vi "Get_Weld_History_Repeated_webserver.vi"() -> ()   [LabVIEW 2017]
uses:
  Generic_Common/Webserver/html_report_cluster.ctl
  <vilib>/httpClient/LabVIEWHTTPClient.lvlib
panel:
  out "vi path":path
  out "Fail":picture
  out "Pass":picture
  out "Iteration Status":bool[](array[boolean])
  out "Grobal Status":bool
  out "Global path":path
  out "Local ini path":path
  out "filename":string
  out "Results Path":path
  in  "Iterations":i32 caption="Iterations (0 to finish:)" min=0
  in  "Resume":bool
  out "error out":errorcluster
  out "key":string
  out "password":string
  out "userid":string
  out "login_url":string
  in  "Delay (ms):":i32
  out "StatusCodeName":string
  out "Session id name":string
  out "logout_url":string
  out "ErrorCode_expected":string
  out "Logout : Header  debug purpose":string
  out "Logout : Body debug purpose":string
  out "Status_message":string
  out "Logo":u16(ring)
  out "Iteration_Indicator":i32
  out "Error code recieved":i32
  out "POST_command":string
  out "Command_url":string
  out "Test case":string
  out "Global ini path":path
  out "Test status":picture
  out "Time elapsed for each iteration":string
  out "DelayBetweenIterations":string
  out "Global_Webserver_Report":string
  out "TestSuite":string
  out "Error Out":errorcluster
  out "Response time":u32[](graph)
  out "Header of reponse for debug pupose":string
  out "Response":string caption="Response from the web server"
  # "AUTOMATION TESTING WEB SERVICES"
  # "TESTING DETAILS FROM INI"
  # "RESPONSE FROM WEBSERVER"
  # "ms"
  # "Webserver \n1. Webserver is being tested in this test case where SC board of ultrasonic welding machine is connected to test PC \t\t  \nSC IP address: 192.168.2.101, url=https://192.168.2.101\t\t\t\t\t\t\t\t\t\t \t\t\t  \n2. Ports used on SC board are as below:\t\t\t\t\t\t\t\t\t\t\t\t\t\t\t\t\t\t\t\t\t  \n   - J103: (Ethernet0) This port connected to UI controller large screen HMI display\trestricted webservices in this port\t\t\t\t\t\t\t\t\t  \n  - J104: (Ethernet1) This port is connected to local area network for accessing the webpage and testing  webserver                                \n  - J112: SC Logs are taken from this port. TeraTerm is configured  to this port so that SC logs are displayed on the screen."
  # "TESTING STATUS"
  # "RESPONSE TIME GRAPH"
  # "GLOBAL TESTING STATUS"
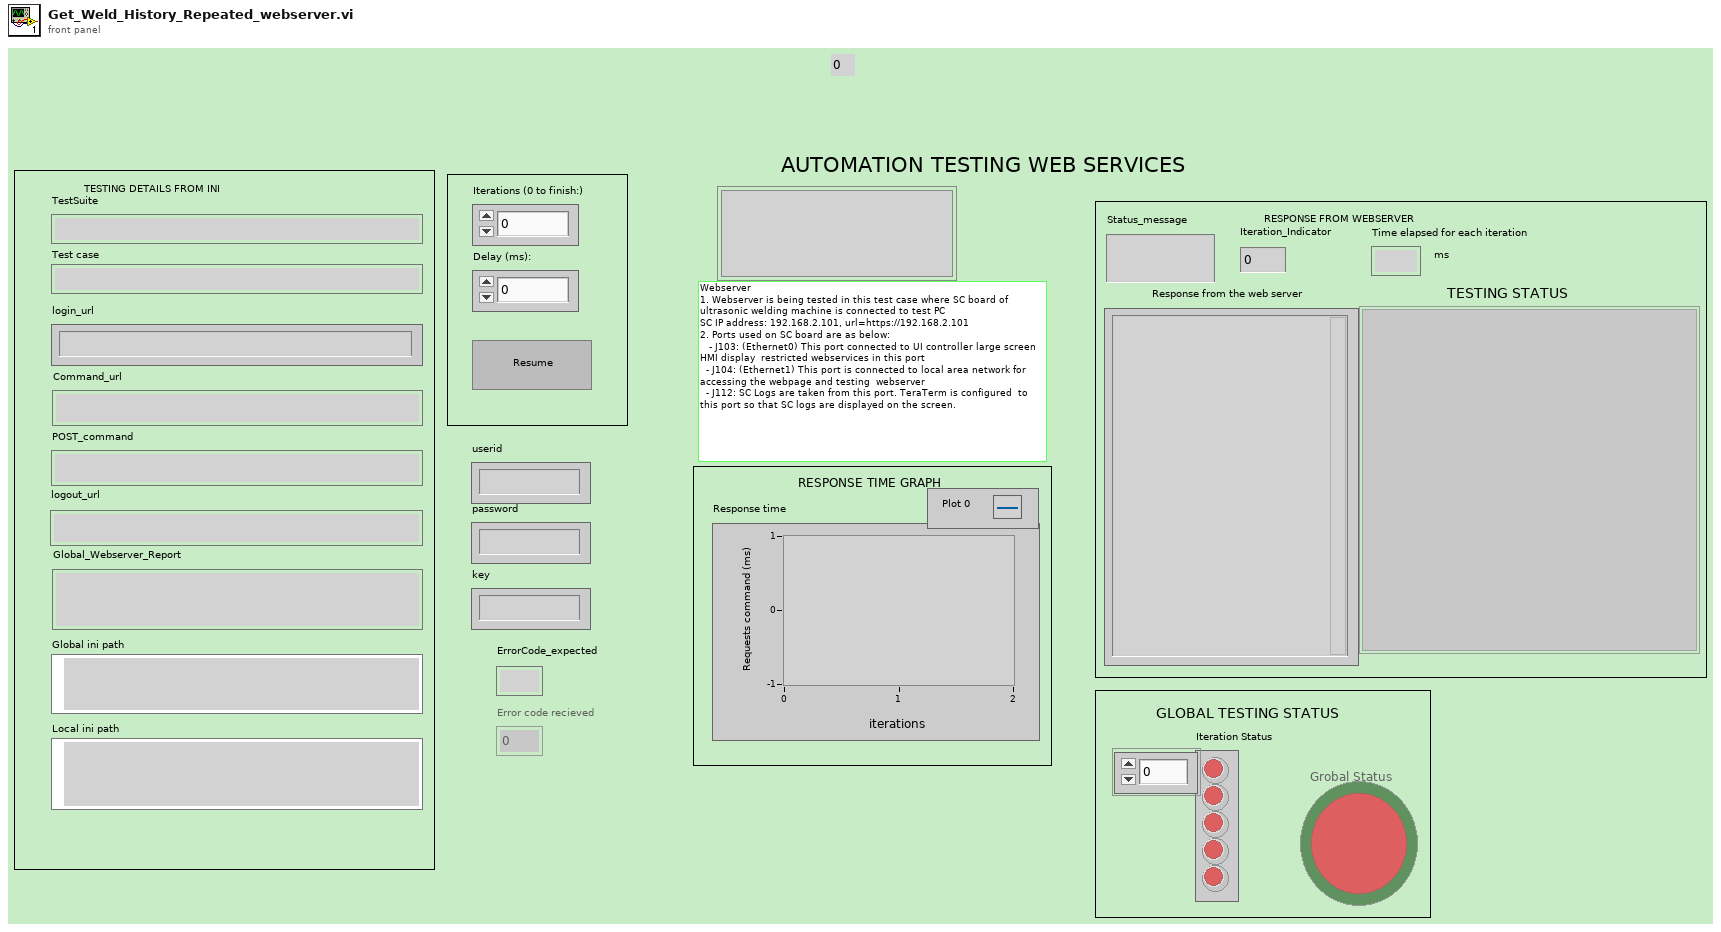
[diagram p1: front panel]
types:
  T1 = enum16{"open", "replace", "create", "open or create", "replace or create", "replace or create with confirmation"}
  T2 = enum8{"Enabled", "Disabled", "Disabled and Grayed Out"}
  T3 = typedef "imagedata.ctl" = cluster{"image type":i32, "image depth":i32, "image":u8[], "mask":u8[], "colors":u32[], "Rectangle":cluster{"left":i16, "top":i16, "right":i16, "bottom":i16}}
  T4 = cluster{"[0]":string, "[1]":string, "[2]":string, "[3]":string, "[4]":string, "[5]":string, "[6]":string, "[7]":string, "[8]":string}
  T5 = cluster{"Server_IP_Address":string, "Server_Port_Number":string, "Sid":string, "StatusCodeName":string, "Global_Webserver_Report":string}
  T6 = cluster{"login_url":string, "userid":string, "password":string, "key":string, "command_url":string, "POST_command":string, "StatusCode_expected":string, "Iterations":string, "DelayBetweenIterations":string, "Timeout":string, "logout_url":string}
  T7 = typedef "html_report_cluster.ctl" = cluster{"Remarks":string, "Verdict":string, "Status Code":i32, "Status Description":string, "JazzDashboardLink":string, "ReprtPath":string, "Timestamp":string, "TestSuite":string, "TestCase":string, "Iterations":i64, "Time taken to execute  test in msec":string, "Delay Between Iterations":i64}
  T8 = typedef "LabVIEWHTTPClient.lvlib/ClientHandle.ctl" = refnum<k1>
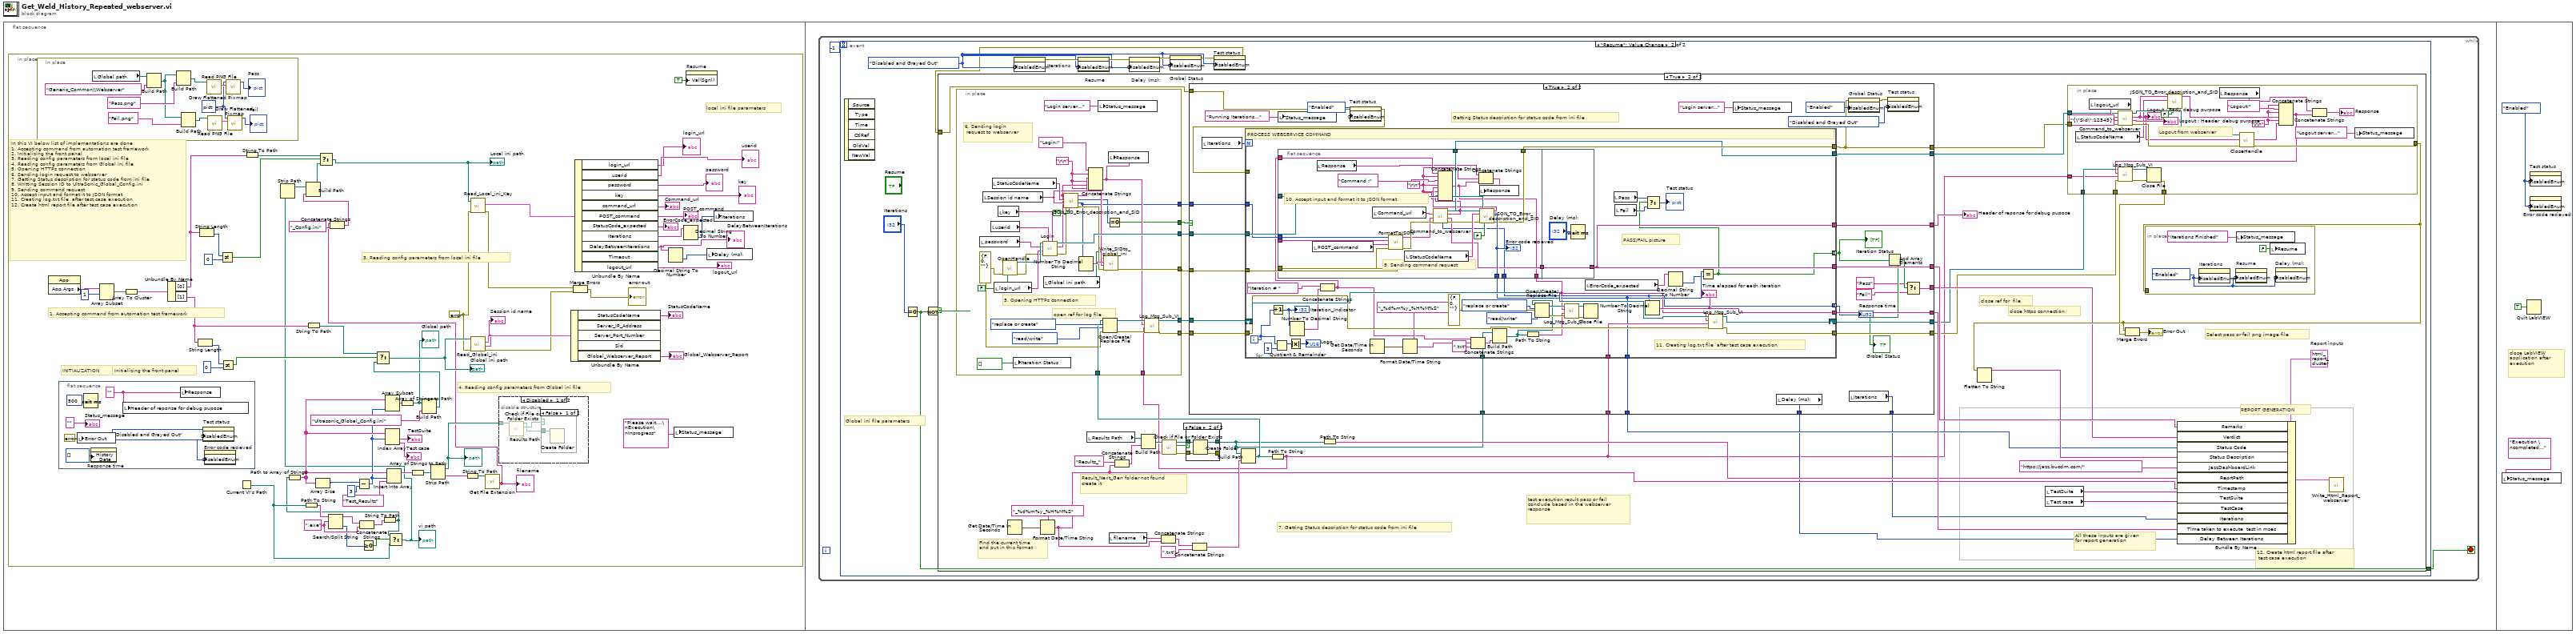
[diagram p0: block diagram]
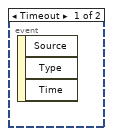
[diagram p4: hidden frame]
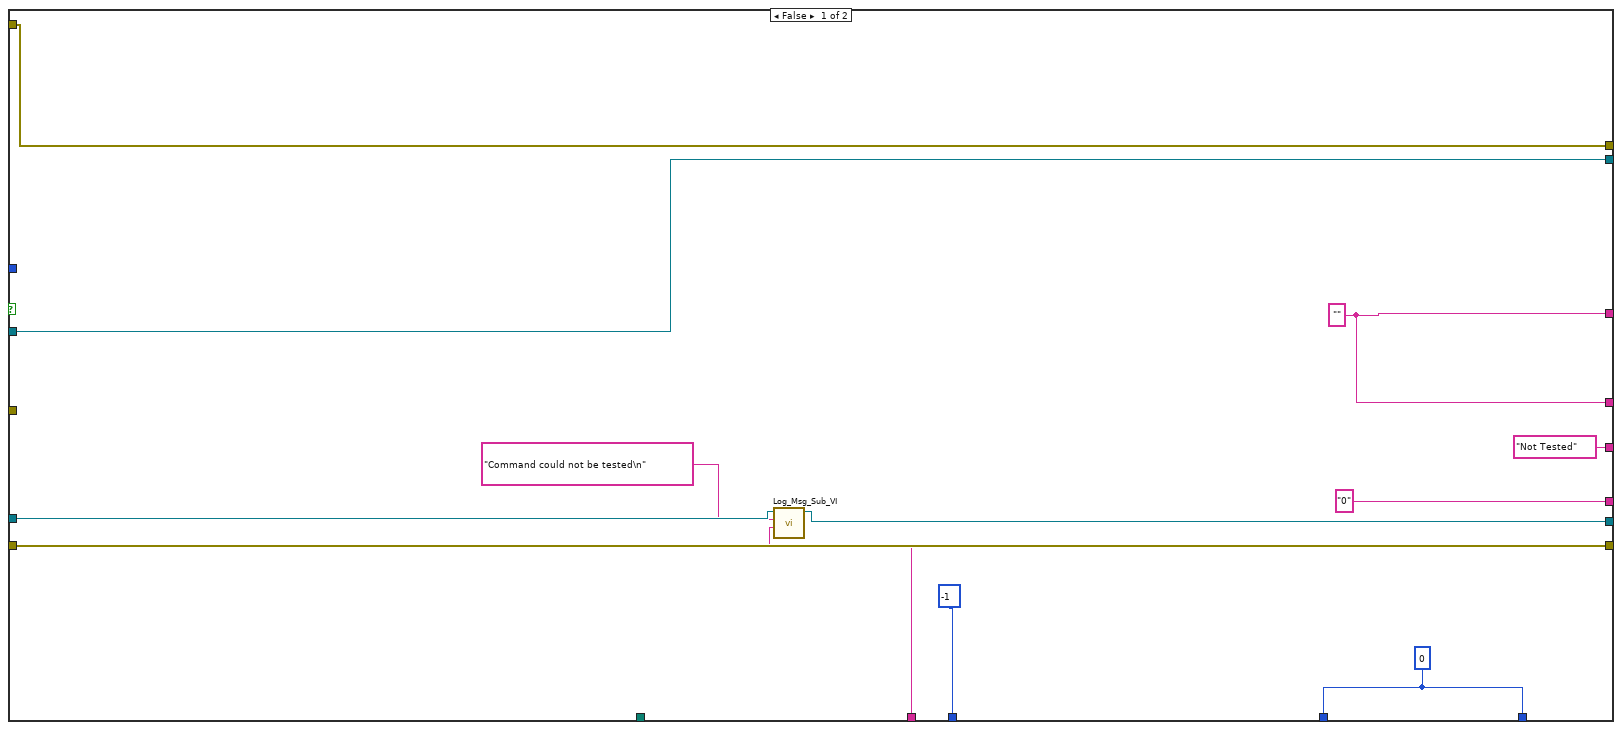
[diagram p6: hidden frame]
diagram:
  n1 = flat-sequence {
    frame #0 {
      n2 = in-place {
        w7 = ".exe" ("search string/char (-)")
        w21 = errorcluster {"status"=FALSE, "code"=0, "source"=""} ("error out")
        # "local ini file parameters"
        # "INITIALIZATION"
        # "4. Reading config parameters from Global ini file"
        # "3. Reading config parameters from local ini file"
        # "2. Initializing the front panel"
        # "1. Accepting command from automation test framework"
        # "In this VI below list of implementations are done\n1. Accepting command from automation test framework\n2. Initializing the front panel\n3. Reading config parameters from local ini file\n4. Reading config parameters from Global ini file\n5. Opening HTTPs connection\n6. Sending login request to webserver\n7. Getting Status description for status code from ini file\n8. Writting Session ID to UltraSonic_Global_Config.ini\n9. Sending command request\n10. Accept input and format it to JSON format\n11. Creating log.txt file  after test case execution\n12. Create html report file after test case execution"
        n3 = in-place {
          w70 = picture data[5B] ("picture")
          n4 = local read "Global path"() -> (w78:path)
          n5 = Build Path(base path=w78, name or relative path="Generic_Common\\Webserver") -> (appended path=w72:path)
          n6 = Build Path(base path=w72, name or relative path="Pass.png") -> (appended path=w76:path)
          n7 = Build Path(base path=w72, name or relative path="Fail.png") -> (appended path=w73:path)
          n8 = call <vilib>:"Read PNG File.vi"("path to PNG file"=w76) -> ("image data"=w80:T3)  [unwired: 8 in, 2 out]
          n9 = call <vilib>:"Read PNG File.vi"("path to PNG file"=w73) -> ("image data"=w75:T3)  [unwired: 8 in, 2 out]
          n10 = call <vilib>:"Draw Flattened Pixmap.vi"("image data"=w80, "picture"=w70) -> ("new picture"=→"Pass":picture)  [unwired: 7 in]
          n11 = call <vilib>:"Draw Flattened Pixmap.vi"("image data"=w75, "picture"=w70) -> ("new picture"=→"Fail":picture)  [unwired: 7 in]
        }
        n12 = property class="App"() -> ("App.Args"=w63:string[])  [unwired: 2 in, 2 out]
        n13 = flat-sequence {
          frame #0 {
            w86 = T2."Disabled and Grayed Out" ("Disabled")
            w91 = ""
            n14 = local write "Error Out"(errorcluster {"status"=FALSE, "code"=0, "source"=""} ("error constant")) -> ()
            n15 = Wait (ms)(milliseconds to wait=u32 500) -> ()  [unwired: 1 out]
            n16 = property on="Response time" class="WFChart (strict)"("History Data"=u32[] []) -> ()  [unwired: 2 in, 2 out]
            n17 = local write "Header of reponse for debug pupose"(w91) -> ()
            n18 = local write "Response"(w91) -> ()
            n19 = property on="Test status" class="Pict"("DisabledEnum"=w86) -> ()  [unwired: 2 in, 2 out]
            n20 = property on="Error code recieved" class="DigNum (strict)"("DisabledEnum"=w86) -> ()  [unwired: 2 in, 2 out]
            "Status_message" <- ""
          }
        }
        n21 = Array Subset "Array Subset"(array=w63, index=1) -> (w64:string[])  [unwired: 1 in]
        n22 = Array To Cluster(array=w64) -> (cluster=w65:T4)
        n23 = Unbundle By Name "Unbundle By Name"(w65) -> ("[0]"=w14:string, "[1]"=w15:string)
        n24 = String Length(string=w15) -> (length=w69:i32)
        n25 = String Length(string=w14) -> (length=w66:i32)
        n26 = Not Equal?(x=w66, y=0) -> (x != y?=w10:bool)
        n27 = Not Equal?(x=w69, y=0) -> (x != y?=w30:bool)
        n28 = Current VI's Path() -> (path=w3:path)
        n29 = String To Path(string=w14) -> (path=w17:path)
        n30 = Path To String(path=w3) -> (string=w9:string)
        n31 = String To Path(string=w15) -> (path=w29:path)
        n32 = Search/Split String(string=w9, search string/char (-)=w7) -> (substring before match=w8:string, offset of match=w4:i32)  [unwired: 1 in, 1 out]
        n33 = Concatenate Strings(w8, w7) -> (w6:string)
        n34 = Greater Or Equal To 0?(x=w4) -> (x >= 0?=w5:bool)
        n35 = String To Path(string=w6) -> (path=w2:path)
        n36 = Path to Array of Strings(0:w2) -> (2:w33:string[])  [unwired: 1 out]
        n37 = Array Size(array=w33) -> (size(s)=w41:i32)
        n38 = Subtract(x=w41, y=3) -> (x-y=w32:i32)
        n39 = Index Array(array=w33, index #1=w32) -> (element #1=→"TestSuite":string, element #2=→"Test case":string)  [unwired: 1 in]
        n40 = Array Subset(array=w33, length=w32) -> (w31:string[])  [unwired: 1 in]
        n41 = Insert Into Array(array=w33, index=w32, new element="Test_Results" ("new element/subarray")) -> (w39:string[])
        n42 = Select(t=w2, s=w5, f=w3) -> (s? t:f=w1:path)
        "vi path" <- w1
        n43 = Strip Path(path=w1) -> (stripped path=w18:path)  [unwired: 1 out]
        n44 = Array of Strings to Path(0:w31) -> (2:w12:path)  [unwired: 1 in]
        "Global path" <- w12
        n45 = Array of Strings to Path(0:w39) -> (2:w40:path)  [unwired: 1 in]
        n46 = Build Path(base path=w12, name or relative path="Ultrasonic_Global_Config.ini") -> (appended path=w23:path)
        n47 = Select(t=w29, s=w30, f=w23) -> (s? t:f=w28:path)
        "Global ini path" <- w28
        n48 = Strip Path(path=w40) -> (stripped path=w36:path, name=w37:string)
        "Results Path" <- w36
        n49 = String To Path(string=w37) -> (path=w38:path)
        n50 = call "Read_Global_ini.vi"("Error In"=w21, "Global ini path"=w28) -> ("Error Out"=w60:errorcluster, "Session id name"=→"Session id name":string, "Global Cluster"=w61:T5)  [unwired: 7 in]
        n51 = call <vilib>:"Get File Extension.vi"("file"=w38) -> ("filename without extension"=w11:string)  [unwired: 6 in, 4 out]
        "filename" <- w11
        n52 = Concatenate Strings(w11, "_Config.ini" ("element")) -> (w20:string)
        n53 = Build Path(base path=w18, name or relative path=w20) -> (appended path=w19:path)
        n54 = Select(t=w17, s=w10, f=w19) -> (s? t:f=w13:path)
        "Local ini path" <- w13
        n55 = call "Read_Local_ini_Key.vi"("Error In"=w21, "Local ini path"=w13) -> ("Error Out"=w59:errorcluster, "cluster"=w57:T6)  [unwired: 8 in]
        n56 = disable-structure shown="Disabled" {
          disable-tunnel: w36 -> [w82 _]
          frame Disabled {
            n57 = call <vilib>:"Check if File or Folder Exists.vi"("path"=w82) -> ("file or folder exists?"=w84:bool, "dup path"=w83:path)  [unwired: 8 in, 1 out]
            n58 = case shown="False" w84 {
              tunnel: w83 -> [w85 _]
              frame False {
                n59 = Create Folder(path (use dialog)=w85) -> ()  [unwired: 2 in, 3 out]
              }
              frame True {
              }
            }
          }
          frame Enabled {
          }
        }
        n60 = Unbundle By Name(w61) -> ("StatusCodeName"=→"StatusCodeName":string, "Global_Webserver_Report"=→"Global_Webserver_Report":string)  [unwired: 3 out]
        n61 = Merge Errors(w59, w60) -> (→"error out":errorcluster)
        n62 = Unbundle By Name(w57) -> ("login_url"=→"login_url":string, "userid"=→"userid":string, "password"=→"password":string, "key"=→"key":string, "command_url"=→"Command_url":string, "POST_command"=→"POST_command":string, "StatusCode_expected"=→"ErrorCode_expected":string, "Iterations"=w53:string, "DelayBetweenIterations"=w52:string, "logout_url"=→"logout_url":string)  [unwired: 1 out]
        "DelayBetweenIterations" <- w52
        n63 = Decimal String To Number(string=w52) -> (number=w47:i32)  [unwired: 2 in, 1 out]
        n64 = local write "Status_message"("Please wait....\nExecution\nInprogress") -> ()
        n65 = Decimal String To Number(string=w53) -> (number=w48:i32)  [unwired: 2 in, 1 out]
        n66 = property on="Resume" class="Bool (strict)"("Val(Sgnl)"=TRUE ("Value (Signaling)")) -> ()  [unwired: 2 in, 2 out]
        n67 = local write "Delay (ms):"(w47) -> ()
        n68 = local write "Iterations"(w48) -> ()
      }
    }
    frame #1 {
      n69 = while {
        stop <- w93 stop-if-true
        n70 = event shown="[1] \"Resume\": Value Change" {
          selector: _ -> [_ _]
          dyn-events: _ -> [_ _]
          timeout: -1 -> [_ _]
          tunnel: [_ w102] -> w93
          event Timeout {
            n71 = event-data() -> ()  [unwired: 1 in, 3 out]
          }
          event "Resume": Value Change {
            w96 = T2."Disabled and Grayed Out" ("Disabled")
            # "Global ini file parameters"
            n72 = event-data() -> ()  [unwired: 1 in, 6 out]
            n73 = Equal To 0?(x="Iterations") -> (x = 0?=w102:bool)
            n74 = Not(x=w102) -> (.not. x?=w101:bool)
            n75 = property on="Iterations" class="DigNum (strict)"("DisabledEnum"=w96) -> (error out=w99:errorcluster)  [unwired: 2 in, 1 out]
            n76 = property on="Resume" class="Bool (strict)"(error in=w99, "DisabledEnum"=w96) -> (error out=w98:errorcluster)  [unwired: 1 in, 1 out]
            n77 = property on="Delay (ms):" class="DigNum (strict)"(error in=w98, "DisabledEnum"=w96) -> (error out=w97:errorcluster)  [unwired: 1 in, 1 out]
            n78 = property on="Grobal Status" class="Bool (strict)"(error in=w97, "DisabledEnum"=w96) -> (error out=w95:errorcluster)  [unwired: 1 in, 1 out]
            n79 = property on="Test status" class="Pict"(error in=w95, "DisabledEnum"=w96) -> (error out=w94:errorcluster)  [unwired: 1 in, 1 out]
            n80 = case shown="True" w101 {
              tunnel: w94 -> [_ w120]
              frame False {
              }
              frame True {
                w146 = T7 {"Remarks"="", "Verdict"="", "Status Code"=0, "Status Description"="", "JazzDashboardLink"="", "ReprtPath"="", "Timestamp"="", "TestSuite"="", "TestCase"="", "Iterations"=0, "Time taken to execute  test in msec"="", "Delay Between Iterations"=1000}  # Report inputs
                # "close https connection"
                # "close ref for  file"
                # "All these inputs are given \nfor report generation"
                # "12. Create html report file after\n test case execution"
                # "7. Getting Status description for status code from ini file"
                # "Select pass or fail png image file"
                # "test execution result pass or fail\nconclude based in the webserver\nresponse"
                # "Find the current time \nand put in this format"
                # "Result_Next_Gen folder not found\ncreate it"
                # "REPORT GENERATION"
                n81 = Get Date/Time In Seconds() -> (seconds since 1Jan1904=w132:timestamp)
                n82 = Format Date/Time String(time format string (%c)="_%d%m%y_%H%M%S", seconds (now)=w132) -> (date/time string=w123:string)  [unwired: 1 in]
                n83 = local read "Results Path"() -> (w130:path)
                n84 = local read "filename"() -> (w131:string)
                n85 = Concatenate Strings("Results_" ("string"), w123) -> (w122:string)
                n86 = Build Path(base path=w130, name or relative path=w122) -> (appended path=w126:path)
                n87 = Concatenate Strings(w131, w123) -> (w128:string)
                n88 = call <vilib>:"Check if File or Folder Exists.vi"("path"=w126) -> ("error out"=w136:errorcluster, "file or folder exists?"=w138:bool, "dup path"=w137:path)  [unwired: 8 in]
                n89 = case shown="False" w138 {
                  tunnel: [w325 w330] -> _
                  tunnel: w137 -> [w326 w329]
                  tunnel: [w326 w328] -> w121
                  tunnel: w136 -> [w325 w327]
                  frame True {
                  }
                  frame False {
                    n90 = Create Folder(path (use dialog)=w329, error in=w327) -> (created path=w328:path, error out=w330:errorcluster)  [unwired: 1 in, 1 out]
                  }
                }
                n91 = Concatenate Strings(w128, ".txt" ("string")) -> (w127:string)
                n92 = Build Path(base path=w121, name or relative path=w127) -> (appended path=w125:path)
                n93 = Path To String(path=w125) -> (string=w103:string)
                n94 = in-place {
                  in-place-border: w125 -> [w180]
                  in-place-border: [w170] -> w117
                  in-place-border: [w163] -> w116
                  in-place-border: [w156] -> w114
                  in-place-border: [w155] -> w113
                  in-place-border: w103 -> [w153]
                  in-place-border: [w152] -> w112
                  in-place-border: [w151] -> w111
                  w159 = "\r\n"
                  w178 = errorcluster {"status"=FALSE, "code"=0, "source"=""} ("error in (no error)")
                  # "6. Sending login\n request to webserver"
                  # "open ref for log file"
                  # "5. Opening HTTPs connection"
                  n95 = local read "password"() -> (w176:string)
                  n96 = local read "Session id name"() -> (w166:string)
                  n97 = local read "userid"() -> (w175:string)
                  n98 = local read "StatusCodeName"() -> (w171:string)
                  n99 = local read "login_url"() -> (w173:string)
                  n100 = local read "key"() -> (w174:string)
                  n101 = call <vilib>:"OpenHandle.vi"("error in (no error)"=w178, "verify server(true)"=FALSE) -> ("client handle out"=w177:T8, "error out"=w172:errorcluster)  [unwired: 12 in]
                  n102 = local write "Iteration Status"(bool[] []) -> ()
                  n103 = call "Login.vi"("key"=w174, "userid"=w175, "Error In"=w172, "Command to webservice"=w173, "password"=w176, "IN HTTPS client handle"=w177) -> ("Error Out"=w168:errorcluster, "Body of reponse"=w160:string, "OUT HTTPS client handle"=w170:T8)  [unwired: 1 in, 2 out]
                  n104 = local read "Global ini path"() -> (w164:path)
                  n105 = call "JSON_TO_Error_description_and_SID.vi"("Sid_present_in_webserver_response"=TRUE, "Error In"=w168, "Session id name"=w166, "Status code name"=w171, "JSON String input"=w160) -> ("Error Out"=w165:errorcluster, "SID"=w152:i32, "status code"=w150:i32, "status_selected"=w162:string)  [unwired: 3 in]
                  n106 = Number To Decimal String(number=w152) -> (decimal integer string=w167:string)  [unwired: 1 in]
                  n107 = Concatenate Strings("Login:" ("string"), w159, w162, w159, w160, w159) -> (w154:string)
                  n108 = local write "Status_message"("Login server..." ("Status_message")) -> ()
                  n109 = Open/Create/Replace File(file path (use dialog)=w180, error in=w178, operation (0:open)=T1."replace or create", access (0:read/write)=enum16{"read/write", "read-only", "write-only"}."read/write") -> (refnum out=w158:refnum<file>, error out=w157:errorcluster)  [unwired: 2 in, 1 out]
                  n110 = call "Write_SIDto_global_ini.vi"("Error In"=w165, "Session id name"=w166, "SID"=w167, "Global ini path"=w164) -> ("Error Out"=w163:errorcluster)  [unwired: 7 in]
                  n111 = Equal To 0?(x=w150) -> (x = 0?=w151:bool)
                  n112 = local write "Response"(w154) -> ()
                  n113 = call "Log_Msg_Sub_VI.vi"("Error In"=w157, "Path for CSV"=w153, "String input"=w154, "refnum in"=w158) -> ("Error Out"=w155:errorcluster, "refnum out"=w156:refnum<file>)  [unwired: 6 in]
                }
                n114 = case shown="True" w111 {
                  tunnel: [w192 w226] -> w147
                  tunnel: [w186 w225] -> w106
                  tunnel: [w194 w224] -> w105
                  tunnel: [w192 w223] -> w142
                  tunnel: ["0" w222] -> w139
                  tunnel: [-1 ("status code") w221] -> w133
                  tunnel: w121 -> [_ w220]
                  tunnel: w120 -> [w193 w200]
                  tunnel: w117 -> [w190 w219]
                  tunnel: w116 -> [_ w218]
                  tunnel: [w193 w208] -> w110
                  tunnel: [w190 w217] -> w115
                  tunnel: w114 -> [w187 w215]
                  tunnel: w113 -> [w194 w214]
                  tunnel: w103 -> [w184 w213]
                  tunnel: w112 -> [_ w212]
                  tunnel: ["Not Tested" w204] -> w109
                  tunnel: [w183 w202] -> w108
                  tunnel: [w183 w201] -> w107
                  frame False {
                    w183 = 0 ("Delay (ms):")
                    w192 = "" ("Header of response for debug purpose")
                    n115 = call "Log_Msg_Sub_VI.vi"("Path for CSV"=w184, "String input"="Command could not be tested\n", "refnum in"=w187) -> ("refnum out"=w186:refnum<file>)  [unwired: 7 in, 1 out]
                  }
                  frame True {
                    # "Getting Status description for status code from ini file"
                    n116 = local read "Iterations"() -> (w211:i32)
                    n117 = local write "Status_message"("Running Iterations..." ("Status_message")) -> ()
                    n118 = property on="Test status" class="Pict"(error in=w200, "DisabledEnum"=T2."Enabled" ("Disabled")) -> (error out=w199:errorcluster)  [unwired: 1 in, 1 out]
                    n119 = for {
                      N: w211 -> [_]
                      tunnel: [w267] -> w226
                      tunnel: [w258] -> w203 mode=indexing
                      tunnel: w214 -> [w270]
                      tunnel: [w268] -> w224
                      tunnel: [w267] -> w223
                      tunnel: [w266] -> w222
                      tunnel: [w259] -> w221
                      tunnel: w213 -> [w261]
                      tunnel: w220 -> [w257]
                      tunnel: w199 -> [_]
                      tunnel: w219 -> [w242]
                      tunnel: w212 -> [w241]
                      tunnel: w218 -> [w240]
                      tunnel: [w239] -> w208
                      tunnel: [w238] -> w217
                      tunnel: [w228] -> w216 mode=indexing
                      shift-right: [w269] -> w225
                      shift-left: w215 -> [w271]
                      i -> [w263]
                      # "PASS/FAIL picture"
                      # "11. Creating log.txt file  after test case execution"
                      # "PROCESS WEBSERVICE COMMAND"
                      n120 = Increment(x=w263) -> (x+1=w235:i32)
                      "Iteration_Indicator" <- w235
                      n121 = Quotient & Remainder(x=w263, y=3) -> (x-y*floor(x/y)=w264:i32)  [unwired: 1 out]
                      n122 = flat-sequence {
                        tunnel: [w291] -> w260
                        tunnel: [w294] -> w259
                        tunnel: [w290] -> w258
                        tunnel: w242 -> [w285]
                        tunnel: w241 -> [w284]
                        tunnel: w240 -> [w283]
                        tunnel: [w282] -> w239
                        tunnel: [w280] -> _
                        tunnel: [w281] -> w238
                        tunnel: w234 -> [w278]
                        tunnel: [w272] -> w233
                        tunnel: w260 -> [w297]
                        tunnel: [w297] -> w267
                        frame #0 {
                          w274 = "\r\n"
                          # "10. Accept input and format it to JSON format"
                          # "9. Sending command request"
                          n123 = local read "POST_command"() -> (w286:string)
                          n124 = local read "Response"() -> (w273:string)
                          n125 = local read "Command_url"() -> (w289:string)
                          n126 = call "FormatToJSON.vi"("Error In"=w283, "Post_command"=w286, "Sid"=w284) -> ("Error Out"=w288:errorcluster, "POST_command_sid_only"=w280:string, "Final_POST_Command"=w287:string)  [unwired: 6 in]
                          n127 = local read "StatusCodeName"() -> (w293:string)
                          n128 = call "Command_to_webserver.vi"("Error In"=w288, "JSON post command"=w287, "URL Command to Logout"=w289, "https client handle in ref"=w285) -> ("Error Out"=w292:errorcluster, "Header of response for debug purpose"=w291:string, "Body of response"=w276:string, "https client handle out ref"=w281:T8, "Reponse time"=w290:u32)  [unwired: 3 in]
                          n129 = call "JSON_TO_Error_description_and_SID.vi"("Sid_present_in_webserver_response"=FALSE, "Error In"=w292, "Status code name"=w293, "JSON String input"=w276) -> ("Error Out"=w282:errorcluster, "status code"=w294:i32, "status_selected"=w279:string)  [unwired: 4 in, 1 out]
                          "Error code recieved" <- w294
                          n130 = Concatenate Strings(w278, w274, "Command :" ("string"), w274, w279, w274, w276, w274) -> (w272:string)
                          n131 = Concatenate Strings(w273, w274, w272) -> (w275:string)
                          n132 = local write "Response"(w275) -> ()
                        }
                        frame #1 {
                          n133 = Wait (ms)(milliseconds to wait="Delay (ms):") -> ()  [unwired: 1 out]
                        }
                      }
                      n134 = Absolute Value(x=w264) -> (abs(x)=→"Logo":i32)
                      n135 = Number To Decimal String(number=w235) -> (decimal integer string=w236:string)  [unwired: 1 in]
                      n136 = Concatenate Strings("Iteration # " ("string"), w236) -> (w234:string)
                      n137 = Get Date/Time In Seconds() -> (seconds since 1Jan1904=w256:timestamp)
                      n138 = Format Date/Time String(time format string (%c)="_%d%m%y_%H%M%S", seconds (now)=w256) -> (date/time string=w248:string)  [unwired: 1 in]
                      n139 = Concatenate Strings(w234, w248, ".txt" ("string")) -> (w247:string)
                      n140 = Build Path(base path=w257, name or relative path=w247) -> (appended path=w245:path)
                      n141 = Path To String(path=w245) -> (string=w244:string)
                      n142 = Open/Create/Replace File(file path (use dialog)=w245, error in=errorcluster {"status"=FALSE, "code"=0, "source"=""}, operation (0:open)=T1."replace or create", access (0:read/write)=enum16{"read/write", "read-only", "write-only"}."read/write") -> (refnum out=w252:refnum<file>, error out=w250:errorcluster)  [unwired: 2 in, 1 out]
                      n143 = call "Log_Msg_Sub_VI.vi"("Error In"=w250, "Path for CSV"=w244, "String input"=w233, "refnum in"=w252) -> ("Error Out"=w249:errorcluster, "refnum out"=w251:refnum<file>)  [unwired: 6 in]
                      n144 = Close File(refnum=w251, error in=w249) -> ()  [unwired: 2 out]
                      n145 = local read "ErrorCode_expected"() -> (w231:string)
                      n146 = local read "Pass"() -> (w230:picture)
                      n147 = local read "Fail"() -> (w229:picture)
                      n148 = Number To Decimal String(number=w258) -> (decimal integer string=w266:string)  [unwired: 1 in]
                      "Time elapsed for each iteration" <- w266
                      n149 = Decimal String To Number(string=w231) -> (number=w232:i32)  [unwired: 2 in, 1 out]
                      n150 = Equal?(x=w259, y=w232) -> (x = y?=w228:bool)
                      n151 = Select(t=w230, s=w228, f=w229) -> (s? t:f=→"Test status":picture)
                      n152 = call "Log_Msg_Sub_VI.vi"("Error In"=w270, "Path for CSV"=w261, "String input"=w233, "refnum in"=w271) -> ("Error Out"=w268:errorcluster, "refnum out"=w269:refnum<file>)  [unwired: 6 in]
                    }
                    "Iteration Status" <- w216
                    "Response time" <- w203
                    n153 = local write "Status_message"("Login server..." ("Status_message")) -> ()
                    n154 = local read "Delay (ms):"() -> (w201:i32)
                    n155 = property on="Grobal Status" class="Bool (strict)"(error in=w208, "DisabledEnum"=T2."Enabled" ("Disabled")) -> (error out=w197:errorcluster)  [unwired: 1 in, 1 out]
                    n156 = local read "Iterations"() -> (w202:i32)
                    n157 = property on="Test status" class="Pict"(error in=w197, "DisabledEnum"=T2."Disabled and Grayed Out" ("Disabled")) -> ()  [unwired: 1 in, 2 out]
                    n158 = And Array Elements(Boolean array=w216) -> (logical AND=w207:bool)
                    "Grobal Status" <- w207
                    n159 = Select(t="Pass", s=w207, f="Fail") -> (s? t:f=w204:string)
                  }
                }
                "Header of reponse for debug pupose" <- w147
                n160 = Path To String(path=w121) -> (string=w135:string)
                n161 = local read "TestSuite"() -> (w144:string)
                n162 = local read "Test case"() -> (w141:string)
                n163 = in-place {
                  in-place-border: [w321] -> w118
                  in-place-border: w110 -> [w319]
                  in-place-border: w115 -> [w318]
                  in-place-border: w106 -> [w304]
                  in-place-border: w105 -> [w303]
                  in-place-border: [w302] -> w104
                  in-place-border: w103 -> [w299]
                  w310 = "\r\n"
                  # "Logout from webserver"
                  n164 = local read "StatusCodeName"() -> (w312:string)
                  n165 = local read "logout_url"() -> (w320:string)
                  n166 = call "Command_to_webserver.vi"("Error In"=w319, "JSON post command"="{\"Sid\":12345}", "URL Command to Logout"=w320, "https client handle in ref"=w318) -> ("Error Out"=w317:errorcluster, "Header of response for debug purpose"=→"Logout : Header  debug purpose":string, "Body of response"=w309:string, "https client handle out ref"=w315:T8)  [unwired: 3 in, 1 out]
                  "Logout : Body debug purpose" <- w309
                  n167 = call "JSON_TO_Error_description_and_SID.vi"("Sid_present_in_webserver_response"=FALSE, "Status code name"=w312, "JSON String input"=w309) -> ("status_selected"=w311:string)  [unwired: 5 in, 3 out]
                  n168 = local read "Response"() -> (w307:string)
                  n169 = call <vilib>:"CloseHandle.vi"("client handle"=w315, "error in (no error)"=w317) -> ("error out"=w321:errorcluster)  [unwired: 13 in]
                  n170 = Concatenate Strings(w310, "Logout:" ("string"), w310, w311, w310, w309) -> (w305:string)
                  n171 = call "Log_Msg_Sub_VI.vi"("Error In"=w303, "Path for CSV"=w299, "String input"=w305, "refnum in"=w304) -> ("Error Out"=w300:errorcluster, "refnum out"=w301:refnum<file>)  [unwired: 6 in]
                  n172 = Close File(refnum=w301, error in=w300) -> (error out=w302:errorcluster)  [unwired: 1 out]
                  n173 = Concatenate Strings(w307, w305) -> (→"Response":string)
                  n174 = local write "Status_message"("Logout server..." ("Status_message")) -> ()
                }
                n175 = Flatten To String(anything=w118) -> (data string=w134:string)  [unwired: 3 in, 2 out]
                n176 = Merge Errors(w118, w104) -> (→"Error Out":errorcluster)
                n177 = in-place {
                  in-place-border: w118 -> [_]
                  w322 = T2."Enabled" ("Disabled")
                  n178 = property on="Iterations" class="DigNum (strict)"("DisabledEnum"=w322) -> ()  [unwired: 2 in, 2 out]
                  n179 = property on="Resume" class="Bool (strict)"("DisabledEnum"=w322) -> ()  [unwired: 2 in, 2 out]
                  n180 = local write "Status_message"("Iterations Finished" ("Status_message")) -> ()
                  n181 = local write "Resume"(FALSE ("Resume")) -> ()
                  n182 = property on="Delay (ms):" class="DigNum (strict)"("DisabledEnum"=w322) -> ()  [unwired: 2 in, 2 out]
                }
                n183 = Bundle By Name(cluster=w146, "Remarks"=w142, "Verdict"=w109, "Status Code"=w133, "Status Description"=w134, "JazzDashboardLink"="https://jazz.bucclm.com/", "ReprtPath"=w135, "Timestamp"=w123, "TestSuite"=w144, "TestCase"=w141, "Iterations"=w108, "Time taken to execute  test in msec"=w139, "Delay Between Iterations"=w107) -> (w145:T7)
                n184 = call "Write_Html_Report_webserver.vi"("Report inputs"=w145) -> ()  [unwired: 18 in, 1 out]
              }
            }
          }
        }
      }
    }
    frame #2 {
      w331 = T2."Enabled" ("Disabled")
      # "close LabVIEW \napplication after \nexecution"
      n185 = local write "Status_message"("Execution \ncompleted...") -> ()
      n186 = Quit LabVIEW(quit? (T)=TRUE) -> ()
      n187 = property on="Test status" class="Pict"("DisabledEnum"=w331) -> ()  [unwired: 2 in, 2 out]
      n188 = property on="Error code recieved" class="DigNum (strict)"("DisabledEnum"=w331) -> ()  [unwired: 2 in, 2 out]
    }
  }
